vi "set_rawData.vi"(8 "error in (no error)":errorcluster, 10 "rawData":variant, 11 "HGF_NetworkData":refnum<class "HGF_NetworkVisitor.lvclass">) -> (0 "error out":errorcluster, 3 "dup HGF_NetworkData":refnum<class "HGF_NetworkVisitor.lvclass">)   [LabVIEW 2014, in "HGF_BaseClasses.lvlib" / "HGF_NetworkVisitor.lvclass"]
uses:
  HGF_NetworkVisitor.lvclass
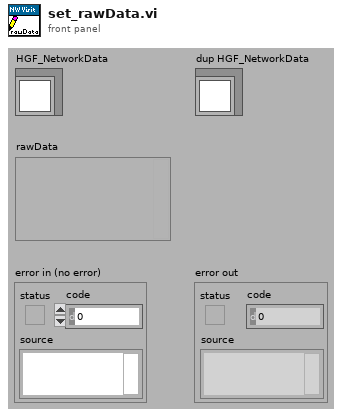
[diagram p1: front panel]
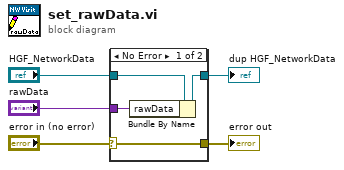
[diagram p0: block diagram]
diagram:
  n1 = case shown="No Error" "error in (no error)" {
    selector: "error in (no error)" -> [w9 w10]
    tunnel: [w9 w10] -> w4
    tunnel: [w7 w11] -> w2
    tunnel: "HGF_NetworkData" -> [w8 w11]
    tunnel: "rawData" -> [w6 _]
    frame No Error {
      n2 = Bundle By Name(cluster=w8, "rawData"=w6) -> (w7:refnum<class "HGF_NetworkVisitor.lvclass">)
    }
    frame Error {
    }
  }
  "error out" <- w4
  "dup HGF_NetworkData" <- w2
